vi "D.vi"(8 "change time":dbl, 9 "D gain":dbl, 10 "prev error":dbl, 11 "error":dbl) -> (1 "output":dbl)   [LabVIEW 2009]
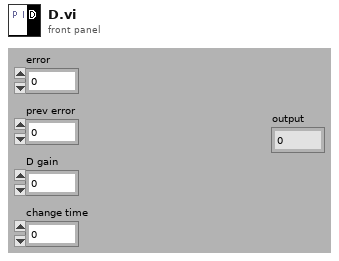
[diagram p1: front panel]
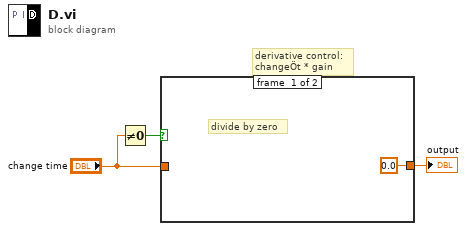
[diagram p0: block diagram]
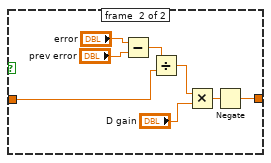
[diagram p2: hidden frame]
diagram:
  # "derivative control:\nchangeÖt * gain"
  n1 = Not Equal To 0?(x="change time") -> (x != 0?=w1:bool)
  n2 = case shown="False" w1 {
    tunnel: [0.0 w6] -> w3
    tunnel: "change time" -> [_ w5]
    frame #0 {
      # "divide by zero"
    }
    frame #1 {
      n3 = Subtract(x="error", y="prev error") -> (x-y=w10:dbl)
      n4 = Divide(x=w10, y=w5) -> (x/y=w9:dbl)
      n5 = Multiply(x=w9, y="D gain") -> (x*y=w7:dbl)
      n6 = Negate(x=w7) -> (-x=w6:dbl)
    }
  }
  "output" <- w3
